vi "Reset.vi"(11 "Electrode Panel":refnum<vi>) -> ()   [LabVIEW 2012, in "StimulCtrls.lvlib"]
uses:
  StimulCtrls.lvlib
  UserControl/ElectdPanel.ctl
  UserControl/ElectdTerminal.ctl
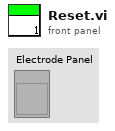
[diagram p1: front panel]
types:
  T1 = enum8{"Enabled", "Disabled", "Disabled and Grayed Out"}
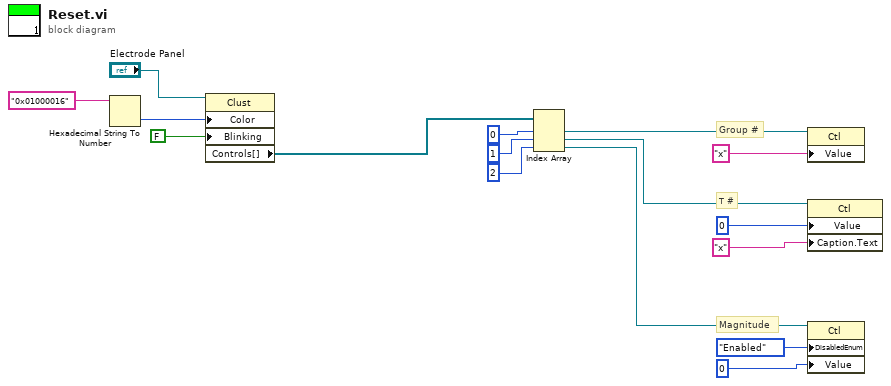
[diagram p0: block diagram]
diagram:
  # "Group #"
  # "Magnitude"
  # "T #"
  n1 = Hexadecimal String To Number(string="0x01000016") -> (number=w8:u32)  [unwired: 2 in, 1 out]
  n2 = property class="Clust"(reference="Electrode Panel", "Color"=w8, "Blinking"=FALSE) -> ("Controls[]"=w1:refnum<vi>[])  [unwired: 1 in, 2 out]
  n3 = Index Array(array=w1, index #1=0 ("index"), index #2=1 ("index"), index #3=2 ("index")) -> (element #1=w16:refnum<vi>, element #2=w15:refnum<vi>, element #3=w14:refnum<vi>)
  n4 = property class="Ctl"(reference=w16, "Value"="x") -> ()  [unwired: 1 in, 2 out]
  n5 = property class="Ctl"(reference=w15, "Value"=0, "Caption.Text"="x") -> ()  [unwired: 1 in, 2 out]
  n6 = property class="Ctl"(reference=w14, "DisabledEnum"=T1."Enabled" ("Disabled"), "Value"=0) -> ()  [unwired: 1 in, 2 out]
